vi "本VI路径.vi"() -> (3 "stripped path":path)   [LabVIEW 2014]
panel:
  out "路径":path
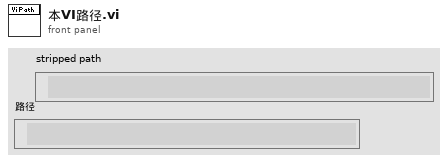
[diagram p1: front panel]
types:
  T1 = enum32{"invalid app kind", "Development System", "Run Time System", "Student Edition", "Embedded LabVIEW", "Evaluation", "Custom"}
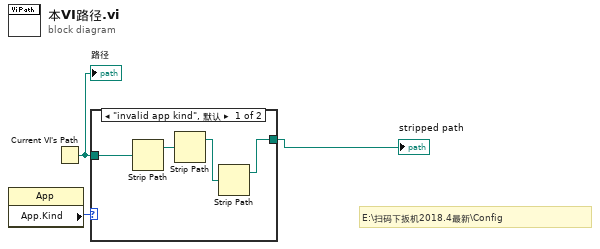
[diagram p0: block diagram]
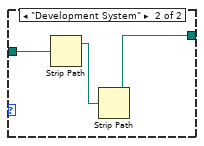
[diagram p2: hidden frame]
diagram:
  # "E:\\扫码下扳机2018.4最新\\Config"
  n1 = property class="App"() -> ("App.Kind"=w3:T1)  [unwired: 2 in, 2 out]
  n2 = Current VI's Path() -> (path=w2:path)
  "路径" <- w2
  n3 = case shown="\"invalid app kind\", 默认" w3 {
    tunnel: w2 -> [w7 w10]
    tunnel: [w4 w8] -> w1
    frame "invalid app kind", Default {
      n4 = Strip Path(path=w7) -> (stripped path=w6:path)  [unwired: 1 out]
      n5 = Strip Path(path=w6) -> (stripped path=w5:path)  [unwired: 1 out]
      n6 = Strip Path(path=w5) -> (stripped path=w4:path)  [unwired: 1 out]
    }
    frame "Development System" {
      n7 = Strip Path(path=w10) -> (stripped path=w9:path)  [unwired: 1 out]
      n8 = Strip Path(path=w9) -> (stripped path=w8:path)  [unwired: 1 out]
    }
  }
  "stripped path" <- w1
